vi "Set Badge.vi"(8 "error in (no error)":errorcluster, 9 "visible":bool, 10 "Badge":T1, 11 "FSM in":refnum<class "FSM.Node.lvclass">) -> (0 "error out":errorcluster, 3 "FSM out":refnum<class "FSM.Node.lvclass">)   [LabVIEW 2015, in "FSM.Node.lvclass"]
uses:
  FSM.Node.lvclass
  Badge.ctl
  FSM.Node.lvclass/FSM.Node.ctl
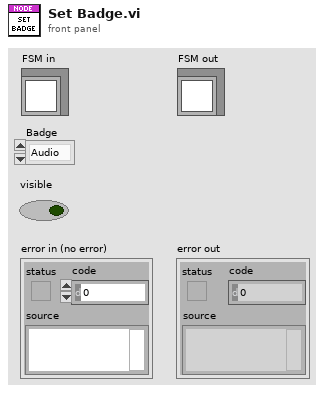
[diagram p1: front panel]
types:
  T1 = typedef "FSM.Node.lvclass/Badge.ctl" = enum16{"Audio", "Visual"}
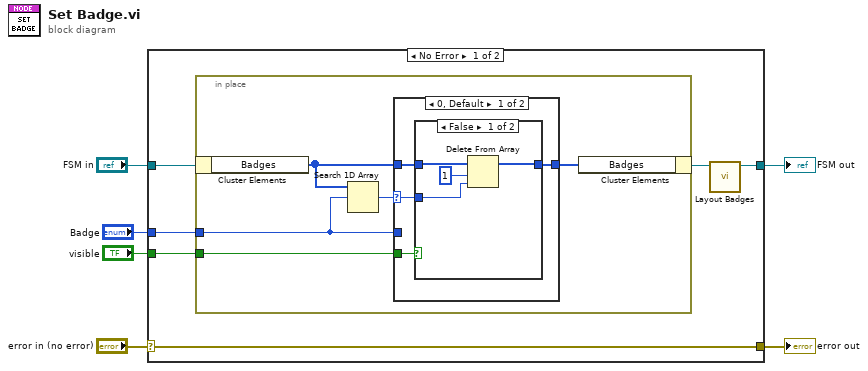
[diagram p0: block diagram]
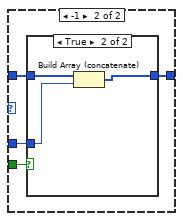
[diagram p3: hidden frame]
diagram:
  n1 = case shown="No Error" "error in (no error)" {
    selector: "error in (no error)" -> [w12 w36]
    tunnel: [w12 w36] -> w5
    tunnel: [w7 w35] -> w3
    tunnel: "FSM in" -> [w10 w35]
    tunnel: "Badge" -> [w11 _]
    tunnel: "visible" -> [w9 _]
    frame No Error {
      n2 = in-place {
        in-place-border: w11 -> [w14]
        in-place-border: w9 -> [w16]
        n3 = in-place-cluster #1(w10) -> ("Badges"=w15:T1[])
        n4 = Search 1D Array(1D array=w15, element=w14) -> (index of element=w17:i32)  [unwired: 1 in]
        n5 = case shown="0, Default" w17 {
          selector: w17 -> [w18 _]
          tunnel: w16 -> [w21 w30]
          tunnel: w15 -> [w19 w29]
          tunnel: w14 -> [_ w28]
          tunnel: [w20 w27] -> w13
          frame 0, Default {
            n6 = case shown="False" w21 {
              tunnel: [w24 w26] -> w20
              tunnel: w19 -> [w25 w26]
              tunnel: w18 -> [w22 _]
              frame False {
                n7 = Delete From Array(array=w25, length=1, index=w22) -> (array with subset deleted=w24:T1[])  [unwired: 1 out]
              }
              frame True {
              }
            }
          }
          frame -1 {
            n8 = case shown="True" w30 {
              tunnel: w29 -> [w31 w34]
              tunnel: w28 -> [_ w33]
              tunnel: [w31 w32] -> w27
              frame False {
              }
              frame True {
                n9 = Build Array (concatenate)(w34, w33) -> (w32:T1[])
              }
            }
          }
        }
        n10 = in-place-cluster #1("Badges"=w13) -> (w8:refnum<class "FSM.Node.lvclass">)
      }
      n11 = call "Layout Badges.vi"("Node in"=w8) -> ("Node out"=w7:refnum<class "FSM.Node.lvclass">)  [unwired: 9 in, 1 out]
    }
    frame Error {
    }
  }
  "error out" <- w5
  "FSM out" <- w3
